vi "Periodic Tasks.vi"(8 "error in":errorcluster) -> ()   [LabVIEW 2014]
doc: "This VI runs in parallel to other tasks. It can contain as many user-defined periodic loops as you need. These can carry out PID or other sorts of timed response."
uses:
  Public/Documents/gsf/Control 1.ctl
  Public/Documents/gsf/Control 2.ctl
  Public/Documents/gsf/Control 3.ctl
  Public/Documents/gsf/Control 4.ctl
  <vilib>/Rock Robotics/WPI/Joystick/WPI_JoystickGetSetRefNum.vi
  <vilib>/Rock Robotics/WPI/RobotDrive/WPI_RobotDriveGetSetRefNum.vi
  <vilib>/addons/control/pid/pid.llb/PID (DBL).vi
  <vilib>/addons/control/pid/NI_PID_pid.lvlib
panel:
  out "Process variable and Setpoint":cluster{"initial PV":dbl, "SP:":dbl}(graph)
  in  "PID gains":T1={"proportional gain (Kc)"=20.0, "integral time (Ti, min)"=0.008, "derivative time (Td, min)"=0.001} {"derivative time (Td, min)" format="%.3f"; "integral time (Ti, min)" format="%.3f"; "proportional gain (Kc)" format="%.3f"}
  out "PV:":dbl(slide)=60.754431603254424 scale=0.0..75.0
  out "SP:":dbl(slide)=43.790849673202615 min=0.0 max=0.0 scale=0.0..75.0
  out "MV:":dbl(slide)=18.78965245852964 scale=-100.0..100.0
  out "Manipulated variable":dbl(graph)
  out "Up":bool
  out "Down":bool
  in  "output range":cluster{"output high":dbl, "output low":dbl}={"output high"=100.0, "output low"=-100.0} {"output low" format="%.2f"; "output high" format="%.2f"}
  out "In Range?":bool
  in  "lower limit":T2
  in  "upper limit":T3
  in  "step inches":T4=25.0 format="%#_13g"
  out "Motor Speed (-1 to 1)":dbl(slide) scale=-1.0..1.0
  in  "Reset Encoder?":bool
  out "Encoder Direction":string
  in  "Stop motor":bool
  out "Encoder Distance":dbl
  in  "y":T5=1023.0 format="%#_13g"
  out "x .and. y?":bool
  out "element":dbl
  in  "Manul drive offset":dbl
  in  "x":dbl=1.0 format="%#_13g"
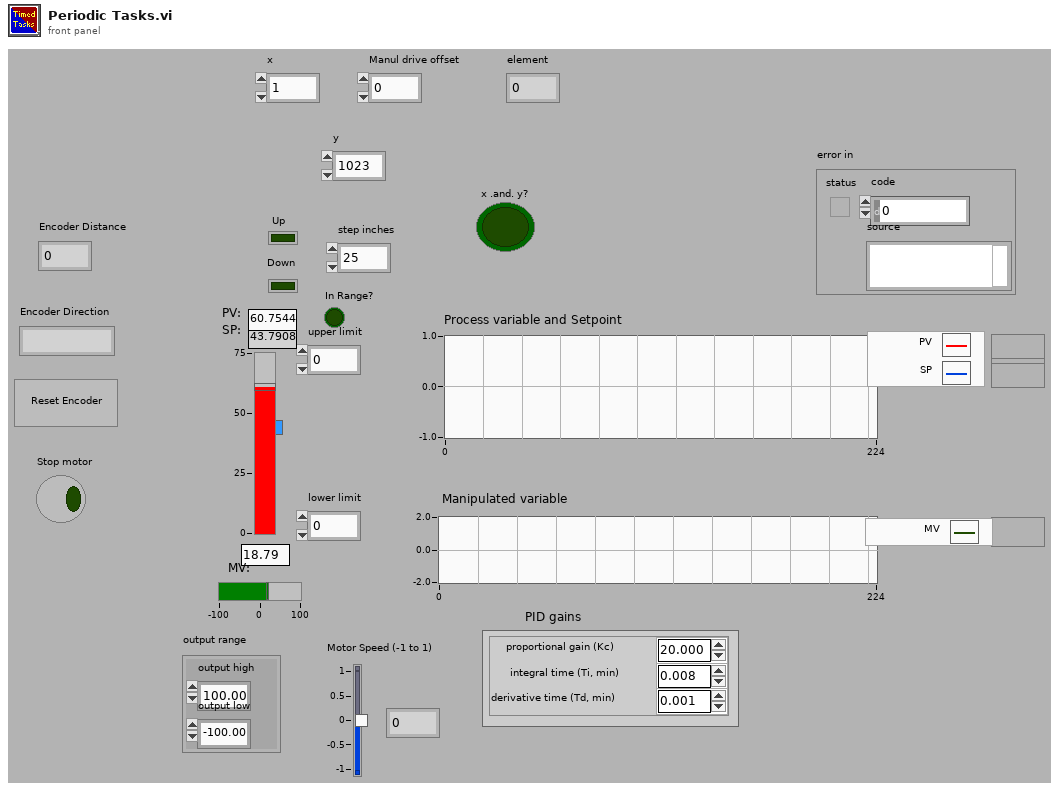
[diagram p1: front panel]
types:
  T1 = cluster{"proportional gain (Kc)":dbl, "integral time (Ti, min)":dbl, "derivative time (Td, min)":dbl}
  T2 = typedef "Control 4.ctl" = dbl
  T3 = typedef "Control 3.ctl" = dbl
  T4 = typedef "Control 2.ctl" = dbl
  T5 = typedef "Control 1.ctl" = dbl
  T6 = typedef "WPI_JoystickDevRef.ctl" = cluster{"Device":T7}
  T7 = typedef "WPI_JoystickDeviceEnum.ctl" = enum16{"USB 0", "USB 1", "USB 2", "USB 3", "USB 4", "USB 5"}
  T8 = typedef "WPI_RobotDriveDevRef.ctl" = cluster{"DevStatus":errorcluster, "Motors[]":T9[], "Square Inputs":bool, "Max Output":dbl}
  T9 = typedef "WPI_MotorControlDeviceRef.ctl" = cluster{"DeviceStatus":errorcluster, "Type":T10, "PWM":cluster{"Controller":T11, "PWM Channel":T12, "DeadBand":T13}, "CAN":cluster{"Device Number":u8, "Control Mode":T14, "Semaphore":T15, "Max Vout":dbl, "TalonSRX Control Mode":T16}, "Invert":bool, "TransformRef":T17, "InvTransformRef":T17}
  T10 = typedef "WPI_MotorControlType.ctl" = enum16{"PWM", "CAN", "CANTalonSRX"}
  T11 = typedef "FPGA_TypedefDigitalModule.ctl" = enum16{"Controller 1"}
  T12 = typedef "FPGA_DIOPWMChannel.ctl" = enum8{"PWM 0", "PWM 1", "PWM 2", "PWM 3", "PWM 4", "PWM 5", "PWM 6", "PWM 7", "PWM 8", "PWM 9", "PWM MXP 0", "PWM MXP 1", "PWM MXP 2", "PWM MXP 3", "PWM MXP 4", "PWM MXP 5", "PWM MXP 6", "PWM MXP 7", "PWM MXP 8", "PWM MXP 9", "Invalid"}
  T13 = typedef "WPI_PWMDeadband.ctl" = cluster{"Name":string, "maxPositivePwm":i32, "minPositivePwm":i32, "centerPwm":i32, "maxNegativePwm":i32, "minNegativePwm":i32, "angularRange":u16}
  T14 = typedef "WPI_CANJaguar_ControlMode.ctl" = enum8{"Percent VBus", "Current", "Speed", "Position", "Voltage"}
  T15 = typedef "Semaphore RefNum" = refnum<k1>
  T16 = typedef "WPI_CANTalonSRX_APIControlMode.ctl" = enum8{"Percent VBus", "Speed", "Position", "Slave", "Unchanged / Invalid"}
  T17 = typedef "WPI_PWMTransform_ConPane.ctl" = refnum<vi>
  T18 = typedef "WPI_EncoderDevRef.ctl" = cluster{"DevStatus":errorcluster, "EncoderIndex":T19, "CounterIndex":T20, "DistancePerCount":dbl, "Decoding Type":T21}
  T19 = typedef "FPGA_EncoderIdx.ctl" = enum8{"Enc 0", "Enc 1", "Enc 2", "Enc 3", "Enc 4", "Enc 5", "Enc 6", "Enc 7", "Invalid"}
  T20 = typedef "FPGA_CounterCtrSystemIndex.ctl" = enum8{"Ctr 0", "Ctr 1", "Ctr 2", "Ctr 3", "Ctr 4", "Ctr 5", "Ctr 6", "Ctr 7", "Invalid"}
  T21 = typedef "WPI_EncoderType.ctl" = enum16{"1x", "2x", "4x"}
  T22 = typedef "WPI_SwitchDevRef.ctl" = cluster{"DevStatus":errorcluster, "DIO Channel":T23, "Controller":T11, "CntIndex":T20, "Normally Closed":bool}
  T23 = typedef "FPGA_DIOChannel.ctl" = enum8{"DIO 0", "DIO 1", "DIO 2", "DIO 3", "DIO 4", "DIO 5", "DIO 6", "DIO 7", "DIO 8", "DIO 9", "DIO MXP 0", "DIO MXP 1", "DIO MXP 2", "DIO MXP 3", "DIO MXP 4", "DIO MXP 5", "DIO MXP 6", "DIO MXP 7", "DIO MXP 8", "DIO MXP 9", "DIO MXP 10", "DIO MXP 11", "DIO MXP 12", "DIO MXP 13", "DIO MXP 14", "DIO MXP 15", "Invalid"}
  T24 = cluster{"JoystickDevRef":T6, "RobotDriveDevRef":T8}
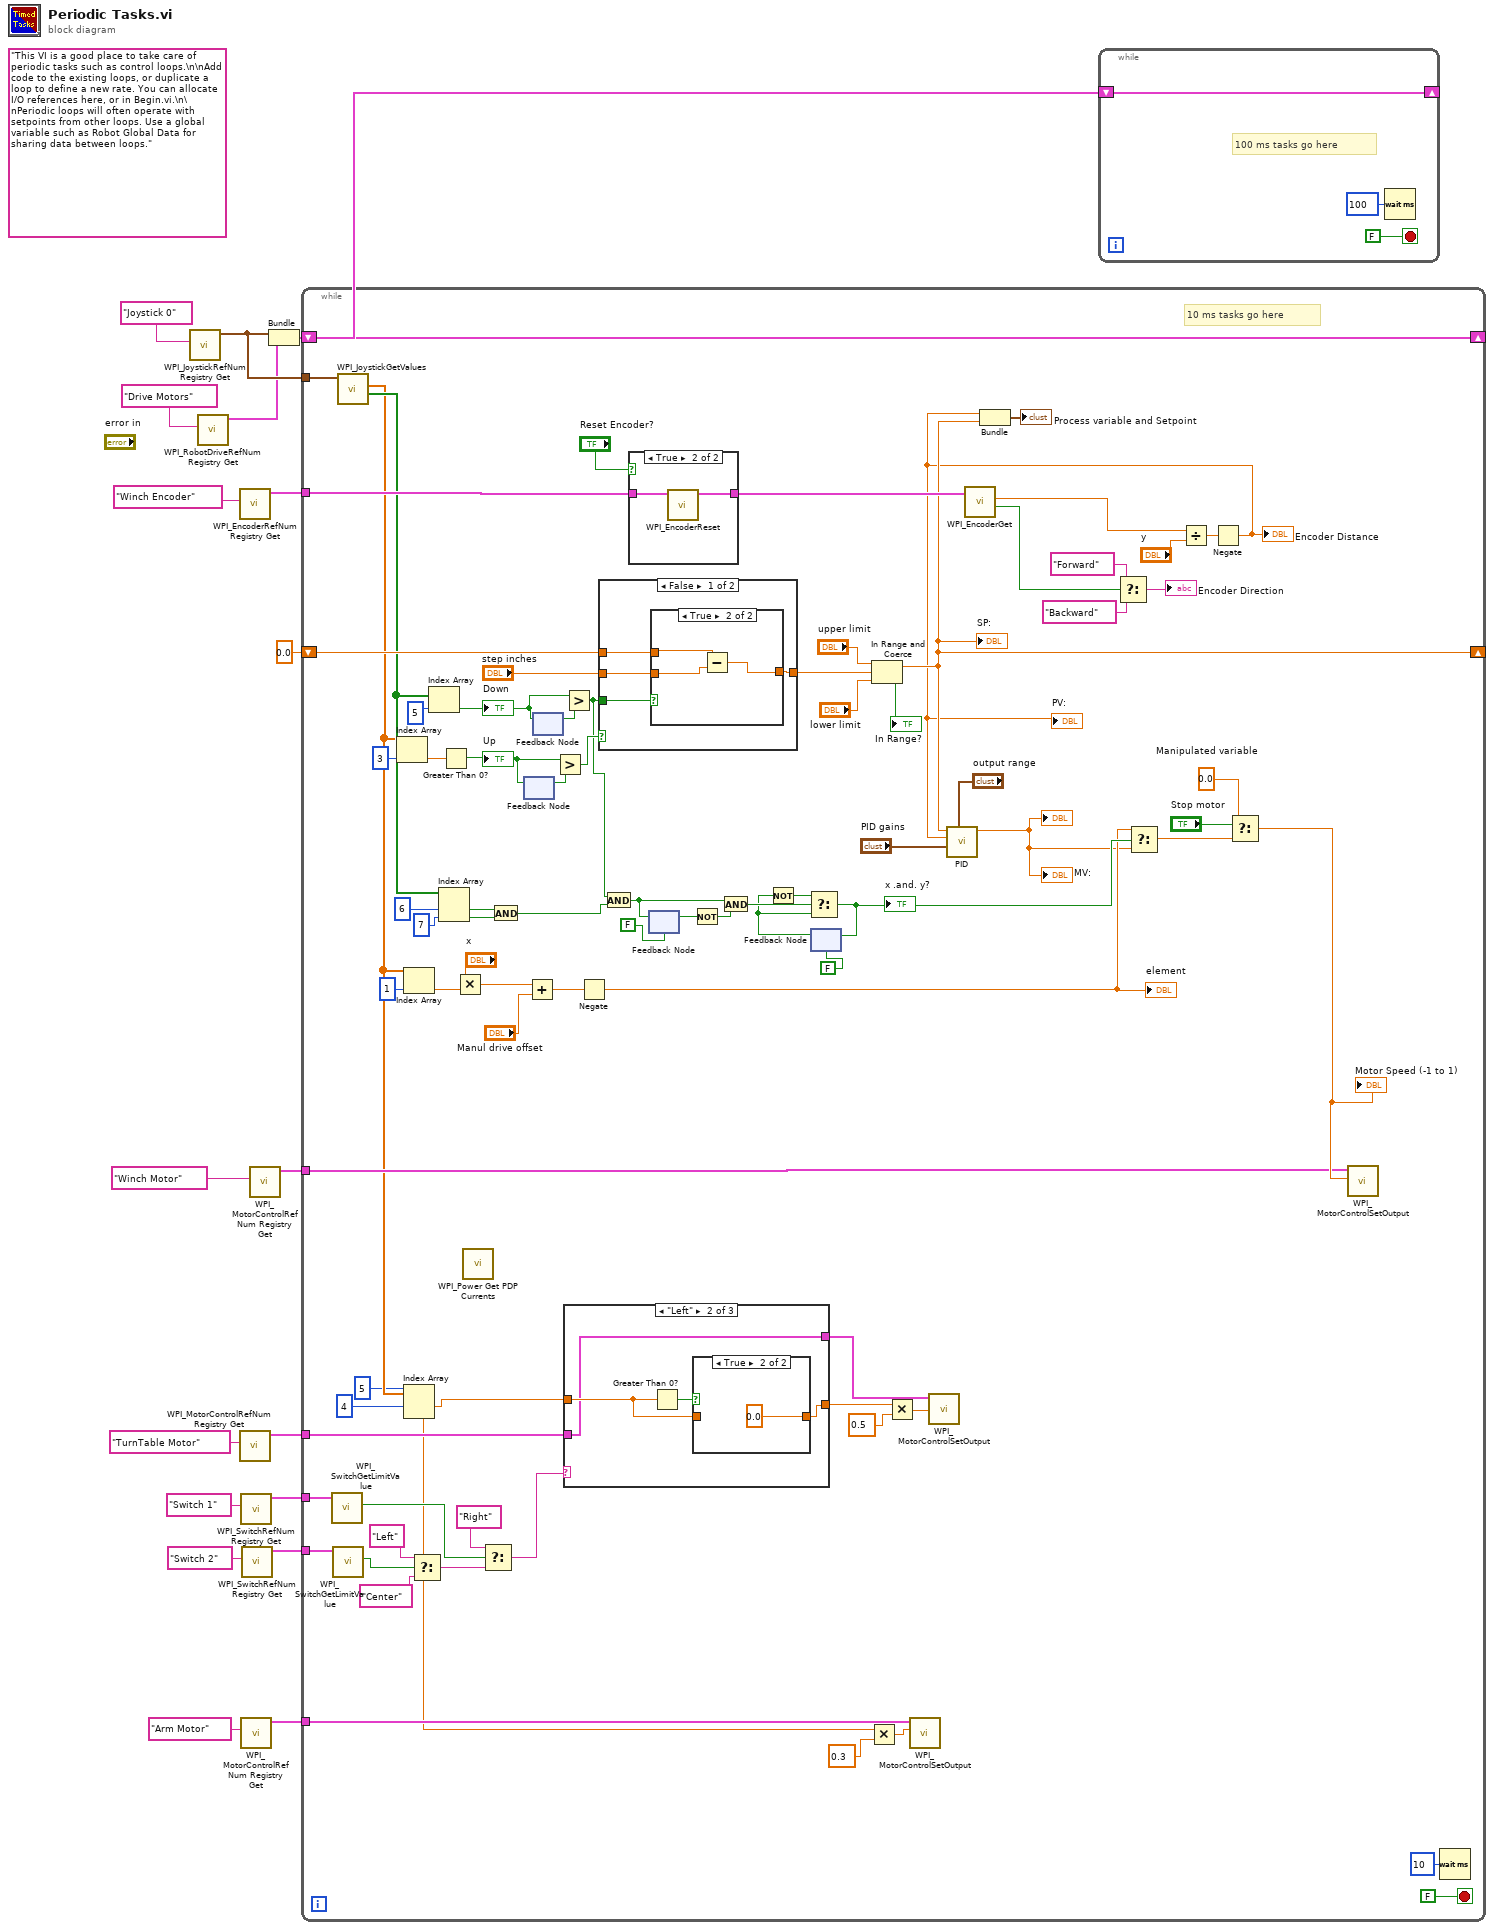
[diagram p0: block diagram]
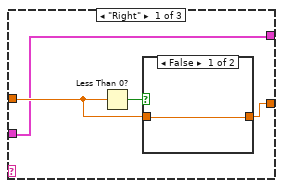
[diagram p2: hidden frame]
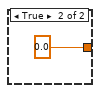
[diagram p3: hidden frame]
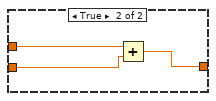
[diagram p8: hidden frame]
diagram:
  (unwired) "This VI is a good place to take care of periodic tasks such as control loops.\n\nAdd code to the existing loops, or duplicate a loop to define a new rate. You can allocate I/O references here, or in Begin.vi.\n\nPeriodic loops will often operate with setpoints from other loops. Use a global variable such as Robot Global Data for sharing data between loops."
  n1 = call <vilib>:"WPI_JoystickRefNum Registry Get.vi"("refnum name"="Joystick 0") -> ("JoystickDevRef"=w17:T6)  [unwired: 1 in, 9 out]
  n2 = call <vilib>:"WPI_RobotDriveRefNum Registry Get.vi"("refnum name"="Drive Motors") -> ("RobotDriveDevRef"=w11:T8)  [unwired: 1 in, 9 out]
  n3 = call <vilib>:"WPI_EncoderRefNum Registry Get.vi"("refnum name"="Winch Encoder") -> ("EncoderDevRef"=w13:T18)  [unwired: 9 in, 1 out]
  n4 = call <vilib>:"WPI_MotorControlRefNum Registry Get.vi"("refnum name"="TurnTable Motor") -> ("MotorControlDevRef"=w6:T9)  [unwired: 9 in, 1 out]
  n5 = call <vilib>:"WPI_SwitchRefNum Registry Get.vi"("refnum name"="Switch 1") -> ("SwitchDevRef"=w1:T22)  [unwired: 9 in, 1 out]
  n6 = call <vilib>:"WPI_MotorControlRefNum Registry Get.vi"("refnum name"="Arm Motor") -> ("MotorControlDevRef"=w5:T9)  [unwired: 9 in, 1 out]
  n7 = call <vilib>:"WPI_SwitchRefNum Registry Get.vi"("refnum name"="Switch 2") -> ("SwitchDevRef"=w2:T22)  [unwired: 9 in, 1 out]
  n8 = call <vilib>:"WPI_MotorControlRefNum Registry Get.vi"("refnum name"="Winch Motor") -> ("MotorControlDevRef"=w16:T9)  [unwired: 9 in, 1 out]
  n9 = Bundle("JoystickDevRef"=w17, "RobotDriveDevRef"=w11) -> (w12:T24)  [unwired: 1 out]
  n10 = while {
    shift-right: [w72] -> _
    shift-left: w12 -> [w72]
    tunnel: w13 -> [w78]
    shift-right: [w76] -> _
    shift-left: 0.0 ("upper limit") -> [w77]
    tunnel: w16 -> [w73]
    tunnel: w17 -> [w71]
    tunnel: w6 -> [w27]
    tunnel: w5 -> [w25]
    tunnel: w2 -> [w36]
    tunnel: w1 -> [w35]
    stop <- FALSE stop-if-true
    # "10 ms tasks go here"
    n11 = call <vilib>:"WPI_SwitchGetLimitValue.vi"("SwitchDevRef"=w35) -> ("Switch Pressed"=w34:bool)  [unwired: 8 in, 2 out]
    n12 = call <vilib>:"WPI_SwitchGetLimitValue.vi"("SwitchDevRef"=w36) -> ("Switch Pressed"=w33:bool)  [unwired: 8 in, 2 out]
    n13 = call <vilib>:"WPI_JoystickGetValues.vi"("JoystickDevRef"=w71) -> ("Buttons"=w65:bool[], "Axes"=w40:dbl[])  [unwired: 6 in, 3 out]
    n14 = Index Array(array=w40, index=3) -> (element=w70:dbl)
    n15 = Index Array(array=w40, index=1) -> (element=w46:dbl)
    n16 = Index Array(array=w40, index #1=4 ("index"), index #2=5 ("index")) -> (element #1=w28:dbl, element #2=w21:dbl)
    n17 = Select(t="Left", s=w33, f="Center") -> (s? t:f=w37:string)
    n18 = Index Array(array=w65, index=5) -> (element=w88:bool)
    "Down" <- w88
    n19 = Index Array(array=w65, index #1=6 ("index"), index #2=7 ("index")) -> (element #1=w63:bool, element #2=w64:bool)
    n20 = Greater Than 0?(x=w70) -> (x > 0?=w69:bool)
    "Up" <- w69
    n21 = Multiply(x="x", y=w46) -> (x*y=w44:dbl)
    n22 = call <vilib>:"WPI_Power Get PDP Currents.vi"() -> ()  [unwired: 13 in, 3 out]
    n23 = Select(t="Right", s=w34, f=w37) -> (s? t:f=w29:string)
    n24 = And(x=w63, y=w64) -> (x .and. y?=w61:bool)
    n25 = feedback #1() -> (w92:bool)  [unwired: 1 in]
    n26 = feedback-in #1(w69) -> ()
    n27 = Add(x=w44, y="Manul drive offset") -> (x+y=w48:dbl)
    n28 = feedback #2() -> (w91:bool)  [unwired: 1 in]
    n29 = feedback-in #2(w88) -> ()
    n30 = Greater?(x=w69, y=w92) -> (0:w62:bool)
    n31 = Greater?(x=w88, y=w91) -> (0:w47:bool)
    n32 = case shown="\"Left\"" w29 {
      tunnel: w28 -> [w105 w111 w116]
      tunnel: w27 -> [w104 w110 w115]
      tunnel: [w104 w110 w115] -> w26
      tunnel: [w103 w109 w116] -> w23
      frame "Right" {
        n33 = Less Than 0?(x=w105) -> (x < 0?=w106:bool)
        n34 = case shown="False" w106 {
          tunnel: w105 -> [w107 _]
          tunnel: [w107 0.0] -> w103
          frame False {
          }
          frame True {
          }
        }
      }
      frame "Left" {
        n35 = Greater Than 0?(x=w111) -> (x > 0?=w112:bool)
        n36 = case shown="True" w112 {
          tunnel: w111 -> [w113 _]
          tunnel: [w113 0.0] -> w109
          frame False {
          }
          frame True {
          }
        }
      }
      frame "Center ", Default {
      }
    }
    n37 = Negate(x=w48) -> (-x=w45:dbl)
    "element" <- w45
    n38 = case shown="False" w62 {
      tunnel: w77 -> [w123 w130]
      tunnel: [w122 w129] -> w97
      tunnel: "step inches" -> [w121 w128]
      tunnel: w47 -> [w120 _]
      frame False {
        n39 = case shown="True" w120 {
          tunnel: [w124 w127] -> w122
          tunnel: w123 -> [w124 w126]
          tunnel: w121 -> [_ w125]
          frame False {
          }
          frame True {
            n40 = Subtract(x=w126, y=w125) -> (x-y=w127:T3)
          }
        }
      }
      frame True {
        n41 = Add(x=w130, y=w128) -> (x+y=w129:T3)
      }
    }
    n42 = And(x=w47, y=w61) -> (x .and. y?=w60:bool)
    n43 = case shown="True" "Reset Encoder?" {
      tunnel: w78 -> [w117 w119]
      tunnel: [w117 w118] -> w89
      frame False {
      }
      frame True {
        n44 = call <vilib>:"WPI_EncoderReset.vi"("EncoderDevRef"=w119) -> ("EncoderDevRef"=w118:T18)  [unwired: 1 in, 9 out]
      }
    }
    n45 = feedback #3(FALSE) -> (w58:bool)
    n46 = feedback-in #3(w60) -> ()
    n47 = Not(x=w58) -> (.not. x?=w59:bool)
    n48 = And(x=w60, y=w59) -> (x .and. y?=w56:bool)
    n49 = feedback #4(FALSE) -> (w55:bool)
    n50 = Not(x=w55) -> (.not. x?=w53:bool)
    n51 = Select(t=w53, s=w56, f=w55) -> (s? t:f=w51:bool)
    "x .and. y?" <- w51
    n52 = feedback-in #4(w51) -> ()
    n53 = Multiply(x=w21, y=0.3) -> (x*y=w19:dbl)
    n54 = In Range and Coerce(upper limit="upper limit", x=w97, lower limit="lower limit") -> (coerced(x)=w76:T3, In Range?=→"In Range?":bool)
    "SP:" <- w76
    n55 = Multiply(x=w23, y=0.5) -> (x*y=w22:dbl)
    n56 = call <vilib>:"WPI_MotorControlSetOutput.vi"("Output"=w19, "MotorControlDevRef"=w25) -> ()  [unwired: 7 in, 3 out]
    n57 = call <vilib>:"WPI_MotorControlSetOutput.vi"("Output"=w22, "MotorControlDevRef"=w26) -> ()  [unwired: 7 in, 3 out]
    n58 = call <vilib>:"WPI_EncoderGet.vi"("EncoderDevRef"=w89) -> ("Direction"=w81:bool, "Distance"=w82:dbl)  [unwired: 1 in, 8 out]
    n59 = Select(t="Forward", s=w81, f="Backward") -> (s? t:f=→"Encoder Direction":string)
    n60 = Divide(x=w82, y="y") -> (x/y=w75:T5)
    n61 = Negate(x=w75) -> (-x=w41:T5)
    "PV:" <- w41
    "Encoder Distance" <- w41
    n62 = call-poly <vilib>:"PID.vi"("output range"="output range", "PID gains"="PID gains", "process variable"=w41, "setpoint"=w76) -> ("output"=w42:dbl)  [unwired: 6 in, 1 out]
    "MV:" <- w42
    "Manipulated variable" <- w42
    n63 = Bundle(w41, "upper limit"=w76) -> (→"Process variable and Setpoint":cluster{T5, "upper limit":T3})  [unwired: 1 in]
    n64 = Select(t=w45, s=w51, f=w42) -> (s? t:f=w52:dbl)
    n65 = Select(t=0.0, s="Stop motor", f=w52) -> (s? t:f=w74:dbl)
    "Motor Speed (-1 to 1)" <- w74
    n66 = call <vilib>:"WPI_MotorControlSetOutput.vi"("Output"=w74, "MotorControlDevRef"=w73) -> ()  [unwired: 2 in, 8 out]
    n67 = Wait (ms)(milliseconds to wait=u32 10) -> ()  [unwired: 1 out]
  }
  n68 = while {
    shift-right: [w131] -> _
    shift-left: w12 -> [w131]
    stop <- FALSE stop-if-true
    # "100 ms tasks go here"
    n69 = Wait (ms)(milliseconds to wait=u32 100) -> ()  [unwired: 1 out]
  }
